vi "Stop Core.vi"(10 "final error code":i32, 11 "Mag Lab Measure Interface in":refnum<class "Mag Lab Measure UI.lvclass">) -> (3 "Mag Lab Measure Interface out":refnum<class "Mag Lab Measure UI.lvclass">)   [LabVIEW 2015, in "Mag Lab Measure UI.lvclass"]
uses:
  Mag Lab Measure UI.lvclass
  Mag Lab Measure UI.lvclass/Mag Lab Measure UI.ctl
  Mag Lab Root/Mag Lab Root.lvclass
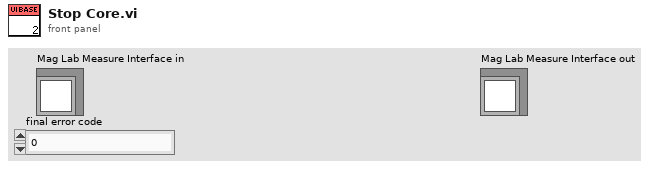
[diagram p1: front panel]
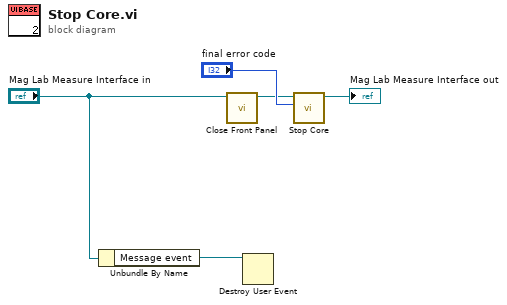
[diagram p0: block diagram]
diagram:
  n1 = Unbundle By Name("Mag Lab Measure Interface in") -> ("Message event"=w2:refnum<user-event>)
  n2 = call-dynamic "Close Front Panel.vi"("Mag Lab Root in"="Mag Lab Measure Interface in") -> ("Mag Lab Root out"=w3:refnum<class "Mag Lab Measure UI.lvclass">)  [unwired: 9 in, 1 out]
  n3 = Destroy User Event(user event=w2) -> ()  [unwired: 1 in, 1 out]
  n4 = call-parent "Stop Core.vi"("final error code"="final error code", "Mag Lab Root in"=w3) -> ("Mag Lab Root out"=→"Mag Lab Measure Interface out":refnum<class "Mag Lab Measure UI.lvclass">)  [unwired: 9 in]
